vi "Mean-SGL.vi"(3 "Data":sgl[](array[numeric])) -> (1 "Mean":sgl)   [LabVIEW 2014]
doc: "Calculate the mean of an array of single precision values. This VI is about 60-70x faster than the double precision, built-in mean routine."
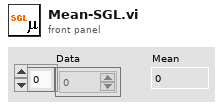
[diagram p1: front panel]
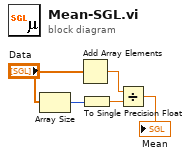
[diagram p0: block diagram]
diagram:
  n1 = Array Size(array="Data") -> (size(s)=w1:i32)
  n2 = Add Array Elements(numeric array="Data") -> (sum=w3:sgl)
  n3 = To Single Precision Float(number=w1) -> (single precision float=w2:sgl)
  n4 = Divide(x=w3, y=w2) -> (x/y=→"Mean":sgl)
